vi "Close_old.vi"(8 "error in":errorcluster, 11 "PPT in":refnum<class "PPT.lvclass">) -> (0 "error out":errorcluster, 3 "PPT out":refnum<class "PPT.lvclass">)   [LabVIEW 2014, in "PPT.lvclass"]
uses:
  PPT.lvclass
  Reusable/Session APIs/Text Communication/Text Device Session.lvclass
  PPT.lvclass/PPT.ctl
  <userlib>/_Session Fwk/Session - Root.lvclass
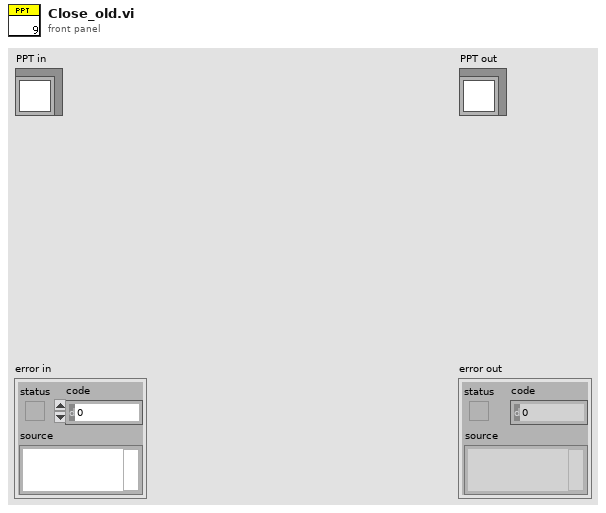
[diagram p1: front panel]
types:
  T1 = typedef "Session - Root.lvclass/Session Handle.ctl" = refnum<data-value>
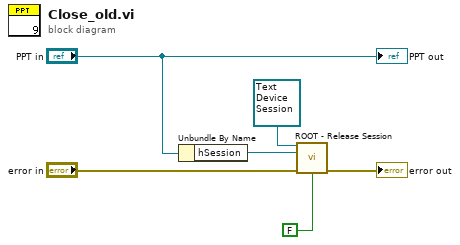
[diagram p0: block diagram]
diagram:
  n1 = Unbundle By Name("PPT in") -> ("hSession"=w5:T1)
  n2 = call <userlib>:"ROOT - Release Session.vi"("OBJ - Session in"=refnum<class "Text Device Session.lvclass"> refnum ("Text Session"), "Session Handle in"=w5, "error in (no error)"="error in", "force destroy? (F)"=FALSE) -> ("error out"=→"error out":errorcluster)  [unwired: 9 in, 2 out]
  "PPT out" <- "PPT in"
